vi "globalVar.vi"() -> ()   [LabVIEW 2024]
panel:
  in  "boardGroup":i32[][](array[numeric])
  in  "boardPiece":i32[][](array[numeric])
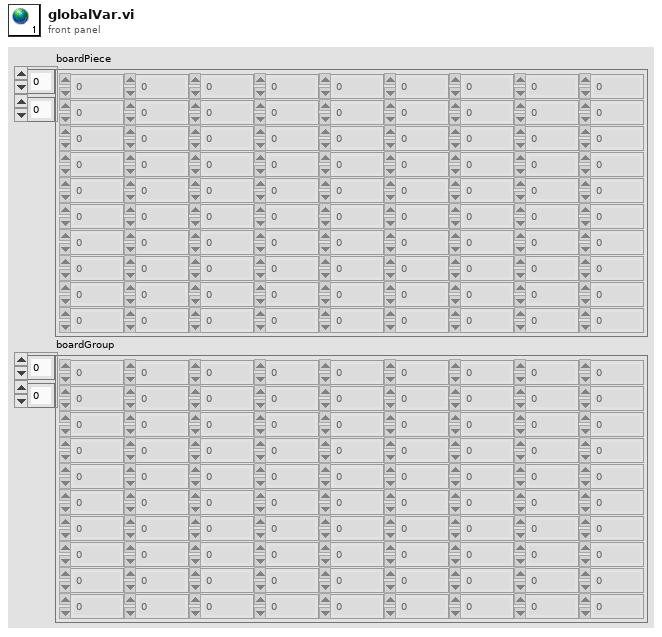
[diagram p1: front panel]
diagram:
